vi "Global-Var-ControlPanel.vi"() -> ()   [LabVIEW 2021]
panel:
  out "CP_broken_nozzle_G":bool
  out "CP_high_temp_G":bool
  out "CP_high_press_tank_G":bool
  out "CP_pump_clogged_G":bool
  out "CP_shiner_low_level_G":bool
  out "CP_soap_low_level_G":bool
  out "CP_water_low_level_G":bool
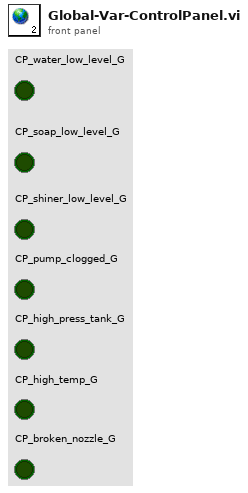
[diagram p1: front panel]
diagram:
